vi "ExSetupROI.vi"() -> ()   [LabVIEW 2010]
uses:
  Open-Close Hardware/CamHandle.vi
panel:
  in  "ADC gain":i32=-1
  in  "ADC port":i32=1
  in  "ADC speed":i32=-2
  out "bit depth":i32
  out "Readout Port":i32
  out "Pixel time":i32
  out "Gain":i32
  out "ADC Speed":u32
  out "error out":errorcluster
  in  "error in (no error)":errorcluster
  in  "Timing Mode":u32(ring)=1 items=["N/A", "Timed Mode/Free run", "Trigger First (only PM)", "Strobed/Ext Sync", "Bulb Mode (PM only)", "Variable Timed mode (PM only)", "Flash Mode (only some PM)"]
  in  "x1":u32=1
  in  "x2":u32=512
  in  "y1":u32=1
  in  "y2":u32=512
  in  "x bin":u32=1
  in  "y bin":u32=1
  in  "min block":u32=2
  in  "Num Min Block":u32=5
  # "User should put in valid ROI"
  # "For Slowest ADC speed set this to -3\nFor Fastest ADC speed set this to -2\nTo use current ADC speed don't  hook up or use -1\notherwise put speed in as kHz"
  # "Note: not all cameras or ADC speeds support \nreadout port. warning message :\nSIWARNING_READOUT_PORT_NOT_SUPPORTED,\t\t  // 5608\n\tSI_LOW_NOISE = 1,\n\tSI_HIGH_CAP = 2,\n\tSI_ELEC_MULT = 3  only available on some cameras"
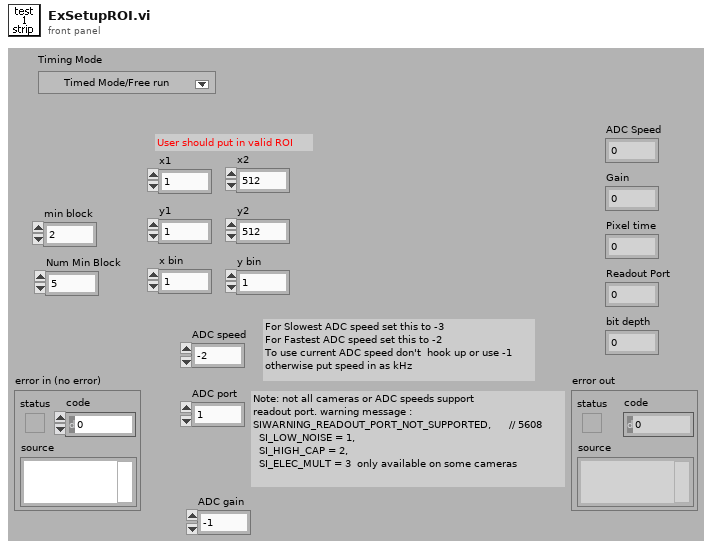
[diagram p1: front panel]
types:
  T1 = cluster{"x1":u32, "x2":u32, "x bin":u32, "y1":u32, "y2":u32, "y bin":u32}
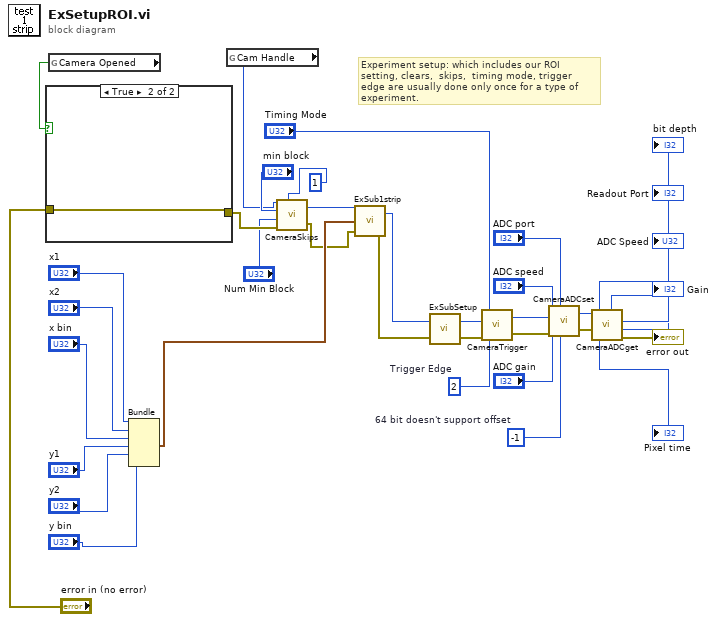
[diagram p0: block diagram]
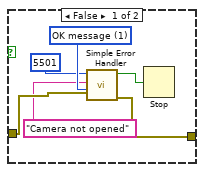
[diagram p2: hidden frame]
diagram:
  w2 = -1  # 64 bit doesn't support offset
  w34 = u32 2  # Trigger Edge
  # "Experiment setup: which includes our ROI setting, clears,  skips,  timing mode, trigger edge are usually done only once for a type of experiment."
  n1 = global read "CamHandle.vi" "Camera Opened"() -> (w33:bool)
  n2 = case shown="True" w33 {
    tunnel: "error in (no error)" -> [w41 w43]
    tunnel: [w40 w43] -> w22
    frame False {
      w42 = u16 1 items=["no dialog", "OK message", "continue or stop message"] ("type of dialog (OK msg:1)")
      n3 = call <vilib>:"Simple Error Handler.vi"("error code (no error:0)"=5501, "error source (\" \")"="Camera not opened", "type of dialog (OK msg:1)"=w42, "error in (no error)"=w41) -> ("error?"=w38:bool, "error out"=w40:errorcluster)  [unwired: 1 in, 3 out]
      n4 = Stop(stop? (T)=w38) -> ()
    }
    frame True {
    }
  }
  n5 = Bundle("x1"="x1", "x2"="x2", "x bin"="x bin", "y1"="y1", "y2"="y2", "y bin"="y bin") -> (w23:T1)  [unwired: 1 in]
  n6 = global read "CamHandle.vi" "Cam Handle"() -> (w15:u32)
  n7 = call <userlib>:"CameraSkips.vi"("Camera Handle"=w15, "Minimum Block Size"="min block", "Number of Minimum blocks"="Num Min Block", "error in"=w22, "Type of Skips"=1) -> ("Camera Handle"=w20:u32, "error out"=w21:errorcluster)
  n8 = call "ExSub1strip.vi"("error in (no error)"=w21, "strip 1"=w23, "Camera Handle"=w20) -> ("error out"=w30:errorcluster, "Camera Handle"=w16:u32)
  n9 = call "ExSubSetup.vi"("error in (no error)"=w30, "Camera Handle"=w16) -> ("error out"=w35:errorcluster, "Camera Handle"=w36:u32)
  n10 = call <userlib>:"CameraTrigger.vi"("error in"=w35, "Trigger Edge"=w34, "Timing Mode"="Timing Mode", "Camera Handle"=w36) -> ("error out"=w32:errorcluster, "Camera Handle"=w31:u32)
  n11 = call <userlib>:"CameraADCset.vi"("ADC offset"=w2, "Read Out port"="ADC port", "error in (no error)"=w32, "ADC Gain"="ADC gain", "ADC Speed"="ADC speed", "Camera Handle"=w31) -> ("error out"=w12:errorcluster, "Camera Handle"=w9:u32)
  n12 = call <userlib>:"CameraADCget.vi"("Camera handle"=w9, "error in (no error)"=w12) -> ("Bit Depth"=→"bit depth":i32, "Pixel Time"=→"Pixel time":i32, "Readout Port"=→"Readout Port":i32, "ADC Speed"=→"ADC Speed":i32, "ADC Gain"=→"Gain":i32, "error out"=→"error out":errorcluster)  [unwired: 2 out]
